vi "Read Data.vi"(8 "error in (no error)":errorcluster, 9 "Data Type (0: FDATA)":i32(ring) items=["FDATA", "RDATA", "SDATA", "FMEM", "SMEM", "SDIV"], 10 "Channel (1)":i32=1, 11 "VISA resource name":refnum<visa-resource-name>) -> (0 "error out":errorcluster, 2 "Data":dbl[](array[numeric]), 3 "VISA resource name out":refnum<visa-resource-name>)   [LabVIEW 2018, in "Keysight PNA Series.lvlib"]
doc: "Reads Measurement data, Memory data, or Normalization Divisor data from the Data Access Map location."
uses:
  Keysight PNA Series.lvlib
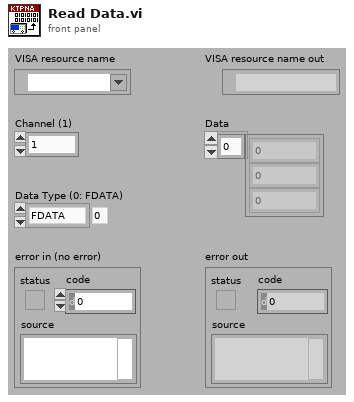
[diagram p1: front panel]
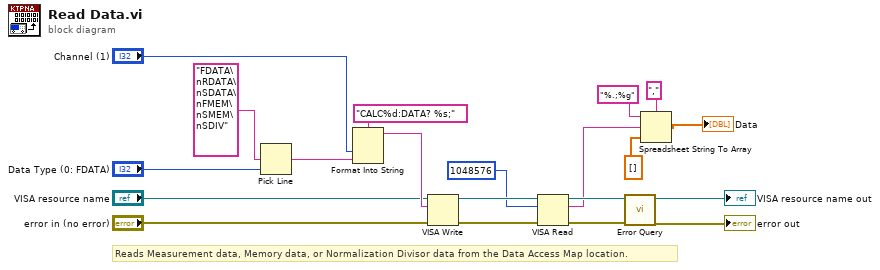
[diagram p0: block diagram]
diagram:
  # "Reads Measurement data, Memory data, or Normalization Divisor data from the Data Access Map location."
  n1 = Pick Line(multi-line string="FDATA\nRDATA\nSDATA\nFMEM\nSMEM\nSDIV", line index="Data Type (0: FDATA)") -> (output string=w16:string)  [unwired: 1 in]
  n2 = Format Into String(format string="CALC%d:DATA? %s;", "Channel (1)", w16) -> (resulting string=w15:string)  [unwired: 2 in, 1 out]
  n3 = VISA Write(VISA resource name="VISA resource name", write buffer=w15, error in (no error)="error in (no error)") -> (VISA resource name out=w8:refnum<visa-resource-name>, error out=w10:errorcluster)  [unwired: 1 out]
  n4 = VISA Read(VISA resource name=w8, byte count=u32 1048576, error in (no error)=w10) -> (VISA resource name out=w7:refnum<visa-resource-name>, read buffer=w3:string, error out=w9:errorcluster)  [unwired: 1 out]
  n5 = call "Error Query.vi"("error in (no error)"=w9, "VISA resource name"=w7) -> ("error out"=→"error out":errorcluster, "VISA resource name out"=→"VISA resource name out":refnum<visa-resource-name>)  [unwired: 6 in, 2 out]
  n6 = Spreadsheet String To Array(delimiter (Tab)=",", format string="%.;%g", spreadsheet string=w3, array type (2D Dbl)=dbl[] [] ("Data")) -> (array=→"Data":dbl[])
